vi "iWorx - Periodic Motion Lab.vi"() -> ()   [LabVIEW 2012]
doc: "This VI is designed to work with myDAQ and the iWorx Light Sensor & Laser to measure periodic tasks."
uses:
  <vilib>/DAQmx/create/channels.llb/DAQmx Create Channel (AI-Voltage-Basic).vi
  <vilib>/DAQmx/configure/timing.llb/DAQmx Timing (Sample Clock).vi
  <vilib>/DAQmx/read.llb/DAQmx Read (Analog 1D Wfm NChan NSamp).vi
panel:
  in  "Analyze":bool caption="Clear Chart"
  in  "Log Info Button":bool
  in  "Stop":bool
  in  "Number of Edges to store":u8=10 min=2
  in  "Channel":u16(ring) items=["Channel 1", "Channel 2"]
  out "Rising Edge Delta t":dbl[](array[numeric]) format="%.3fs"
  out "Beam Break Time":dbl[](array[numeric]) format="%.3fs"
  in  "Threshold":dbl=0.5 format="%.2f V"
  out "Raw Signal":dbl(knob) scale=-5.0..5.0
  in  "Set Up":bool
  in  "Pause Button":bool
  in  "Snapshot":bool
  out "Waveform Chart":waveform(dbl)(graph)
  in  "Clear Chart":bool
  in  "Open Log":bool
  # "Periodic Motion Lab"
  # "Sensor Input"
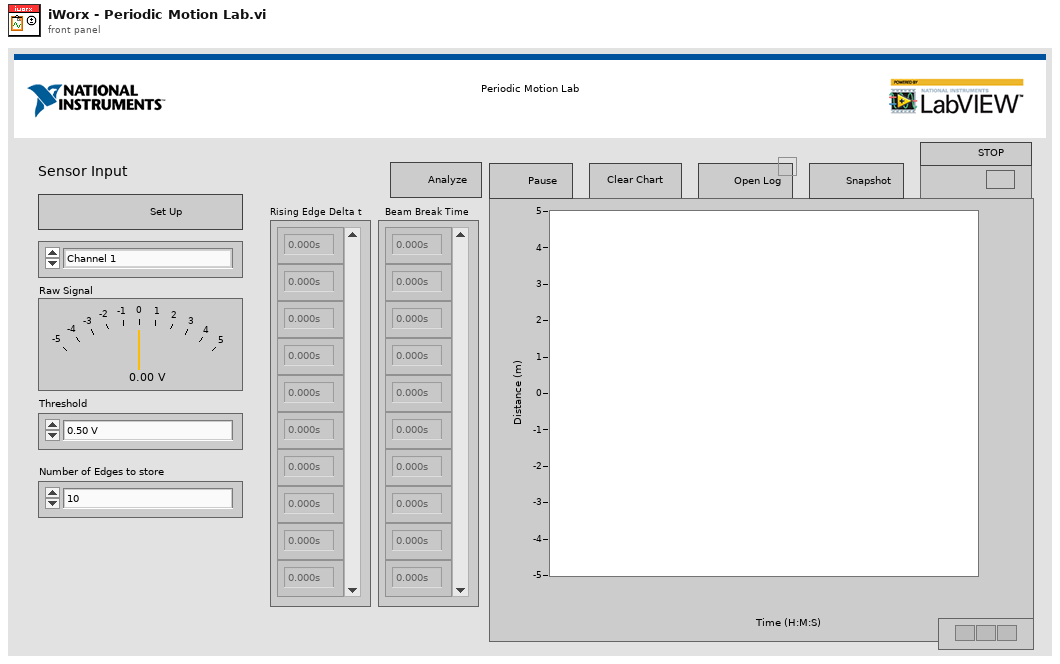
[diagram p1: front panel]
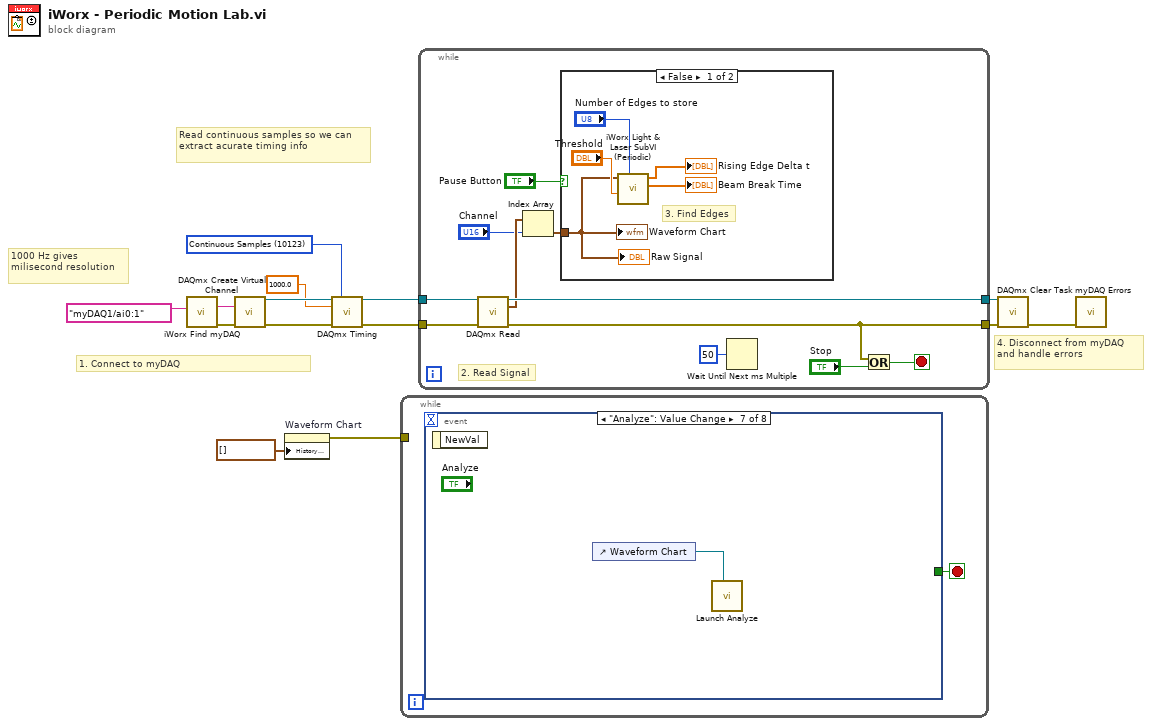
[diagram p0: block diagram]
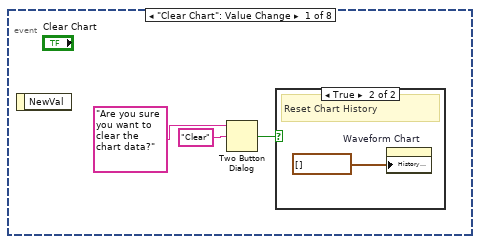
[diagram p2: hidden frame]
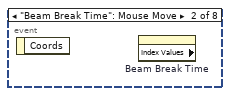
[diagram p4: hidden frame]
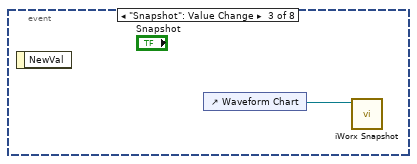
[diagram p5: hidden frame]
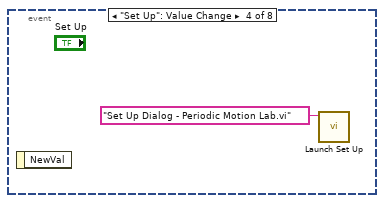
[diagram p6: hidden frame]
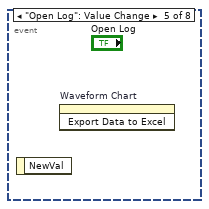
[diagram p7: hidden frame]
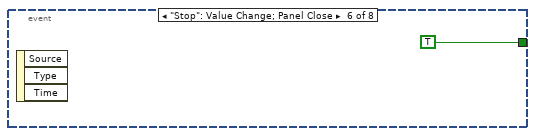
[diagram p8: hidden frame]
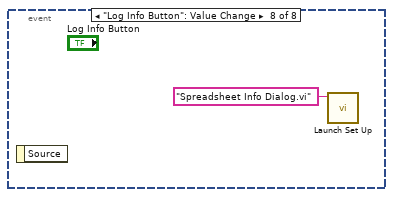
[diagram p9: hidden frame]
diagram:
  w6 = 10123 items=["Finite Samples"=10178, "Continuous Samples"=10123, "Hardware Timed Single Point"=12522] ("sample mode")
  # "4. Disconnect from myDAQ and handle errors"
  # "1. Connect to myDAQ"
  # "1000 Hz gives milisecond resolution"
  # "Read continuous samples so we can extract acurate timing info"
  n1 = call "iWorx Find myDAQ.vi"("Preferred myDAQ (myDAQ1)"=tag "myDAQ1/ai0:1" ("physical channels")) -> ("Error Out"=w4:errorcluster, "DAQmx Physical Channel"=w2:tag)  [unwired: 6 in, 3 out]
  n2 = call-poly <vilib>:"DAQmx Create Virtual Channel.vi"("physical channels"=w2, "error in"=w4) -> ("task out"=w11:refnum<k21>, "error out"=w8:errorcluster)  [unwired: 12 in]
  n3 = property on="Waveform Chart" class="WFChart (strict)"("History Data"=waveform(dbl)[] []) -> (error out=w12:errorcluster)  [unwired: 2 in, 1 out]
  n4 = call-poly <vilib>:"DAQmx Timing.vi"("task/channels in"=w11, "sample mode"=w6, "rate"=1000.0, "error in"=w8) -> ("task out"=w10:refnum<k21>, "error out"=w9:errorcluster)  [unwired: 10 in]
  n5 = while {
    tunnel: w12 -> [_]
    stop <- w15 stop-if-true
    n6 = event shown="[6] \"Analyze\": Value Change" {
      selector: _ -> [_ _ _ _ _ _ _ _]
      dyn-events: _ -> [_ _ _ _ _ _ _ _]
      timeout: _ -> [_ _ _ _ _ _ _ _]
      tunnel: [_ _ _ _ _ TRUE _ _] -> w15
      event "Clear Chart": Value Change {
        n7 = event-data() -> ()  [unwired: 1 in, 1 out]
        n8 = Two Button Dialog(message="Are you sure you want to clear the chart data?", 2:"Clear" ("T button name (\"OK\")")) -> (T button?=w17:bool)  [unwired: 1 in]
        n9 = case shown="True" w17 {
          frame False {
            # "Dialog canceled"
          }
          frame True {
            # "Reset Chart History"
            n10 = property on="Waveform Chart" class="WFChart (strict)"("History Data"=waveform(dbl)[] []) -> ()  [unwired: 2 in, 2 out]
          }
        }
      }
      event "Beam Break Time": Mouse Move {
        n11 = event-data() -> ()  [unwired: 1 in, 1 out]
        n12 = property on="Beam Break Time" class="Arr (strict)" props=["Index Values"]() -> ()  [unwired: 2 in, 3 out]
      }
      event "Snapshot": Value Change {
        n13 = event-data() -> ()  [unwired: 1 in, 1 out]
        n14 = control-ref of="Waveform Chart"() -> (w20:refnum<vi>)
        n15 = call "iWorx Snapshot.vi"("WaveformChart in"=w20) -> ()  [unwired: 10 in, 1 out]
      }
      event "Set Up": Value Change {
        n16 = event-data() -> ()  [unwired: 1 in, 1 out]
        n17 = call "Launch Set Up.vi"("name or relative path"="Set Up Dialog - Periodic Motion Lab.vi") -> ()  [unwired: 9 in, 2 out]
      }
      event "Open Log": Value Change {
        n18 = event-data() -> ()  [unwired: 1 in, 1 out]
        n19 = invoke on="Waveform Chart" class="WFChart (strict)" method="Export Data to Excel"() -> ()  [unwired: 3 in, 3 out]
      }
      event "Stop": Value Change; Panel Close {
        n20 = event-data() -> ()  [unwired: 1 in, 3 out]
      }
      event "Analyze": Value Change {
        n21 = event-data() -> ()  [unwired: 1 in, 1 out]
        n22 = control-ref of="Waveform Chart"() -> (w23:refnum<vi>)
        n23 = call "Launch Analyze.vi"("Chart Ref"=w23) -> ()  [unwired: 9 in, 2 out]
      }
      event "Log Info Button": Value Change {
        n24 = event-data() -> ()  [unwired: 1 in, 1 out]
        n25 = call "Launch Set Up.vi"("name or relative path"="Spreadsheet Info Dialog.vi") -> ()  [unwired: 9 in, 2 out]
      }
    }
  }
  n26 = while {
    tunnel: w10 -> [w35]
    tunnel: [w30] -> w14
    tunnel: w9 -> [w34]
    tunnel: [w32] -> w13
    stop <- w33 stop-if-true
    # "2. Read Signal"
    n27 = call-poly <vilib>:"DAQmx Read.vi"("task/channels in"=w35, "error in"=w34) -> ("task out"=w30:refnum<k21>, "data"=w28:waveform(dbl)[], "error out"=w32:errorcluster)  [unwired: 11 in]
    n28 = Index Array(array=w28, index="Channel") -> (element=w27:waveform(dbl))
    n29 = case shown="False" "Pause Button" {
      tunnel: w27 -> [w39 _]
      frame False {
        # "3. Find Edges"
        n30 = call "iWorx Light & Laser SubVI (Periodic).vi"("# of Timestamps to store (10)"="Number of Edges to store", "Threshold"="Threshold", "Waveform"=w39) -> ("Beam Break Durration (s)"=→"Beam Break Time":dbl[], "Rising Edge Delta t (s)"=→"Rising Edge Delta t":dbl[])  [unwired: 5 in, 2 out]
        "Waveform Chart" <- w39
        "Raw Signal" <- w39
      }
      frame True {
      }
    }
    n31 = Wait Until Next ms Multiple(millisecond multiple=u32 50) -> ()  [unwired: 1 out]
    n32 = Or(x=w32, y="Stop") -> (x .or. y?=w33:bool)
  }
  n33 = call <vilib>:"DAQmx Clear Task.vi"("task in"=w14, "error in"=w13) -> ("error out"=w1:errorcluster)  [unwired: 13 in]
  n34 = call "myDAQ Errors.vi"("error in (no error)"=w1) -> ()  [unwired: 10 in, 1 out]
